vi "Commit DAQ Tags.vi"(8 "error in (no error)":errorcluster, 11 "DAQ State in":T1) -> (0 "error out":errorcluster, 3 "DAQ State out":T1)   [LabVIEW 2018, in "DAQ.lvlib" / "DAQ Write.lvlib"]
uses:
  DAQ Write.lvlib
  Acquisition/Hardware Configuration.ctl
  Acquisition/Task Cluster.ctl
  Tag VIs/Tag FGV Operation Enum.ctl
  Shared Variables/Dynamic Shared Variables.lvlib
  <resource>/objmgr/daqmx.rc
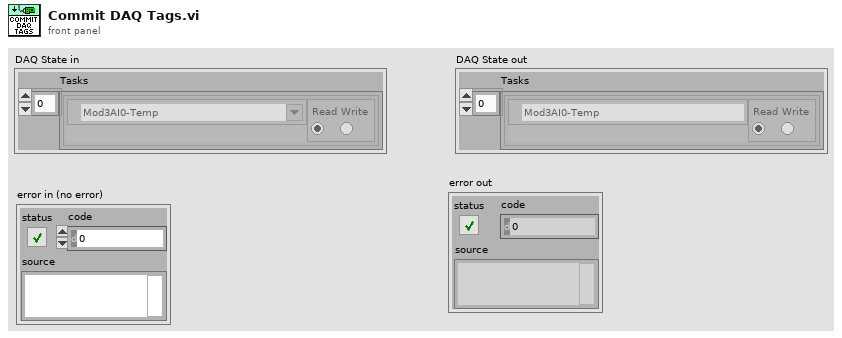
[diagram p1: front panel]
types:
  T1 = typedef "DAQ.lvlib/DAQ Write.lvlib/Hardware Configuration.ctl" = cluster{"Tasks":T2[]}
  T2 = typedef "Task Cluster.ctl" = cluster{"DAQmx Task":refnum<k21>, "Read-Write Radio":enum32{"Read", "Write"}}
  T3 = typedef "Tag FGV Operation Enum.ctl" = enum16{"Init", "Set Notification Queue", "Create Tag", "Commit", "Write Tag (Numeric)", "Write Tag (Boolean)", "Read All Tags", "Read One Tag", "Delete Tag Category", "Set Alarm Parameters (Numeric)", "Set Alarm Parameters (Boolean)", "Enable All Alarms", "Disable All Alarms", "Delete All Tags", "Read Alarms", "Ack Alarm", "Read Alarm Parameters (Numeric)", "Read Alarm Parameters (Boolean)"}
  T4 = enum32{"u32BitField", "bool", "double", "string", "int8", "uint8", "int16", "uint16", "int32", "uint32", "int64", "uint64", "single", "double waveform", "int16 waveform", "array of boolean", "array of int8", "array of uint8", "array of int16", "array of uint16", "array of int32", "array of uint32", "array of int64", "array of uint64", "array of single", "array of double", "array of double waveform", "array of int16 waveform", "array of string", "variant", "timestamp", "fixed point", "custom"}
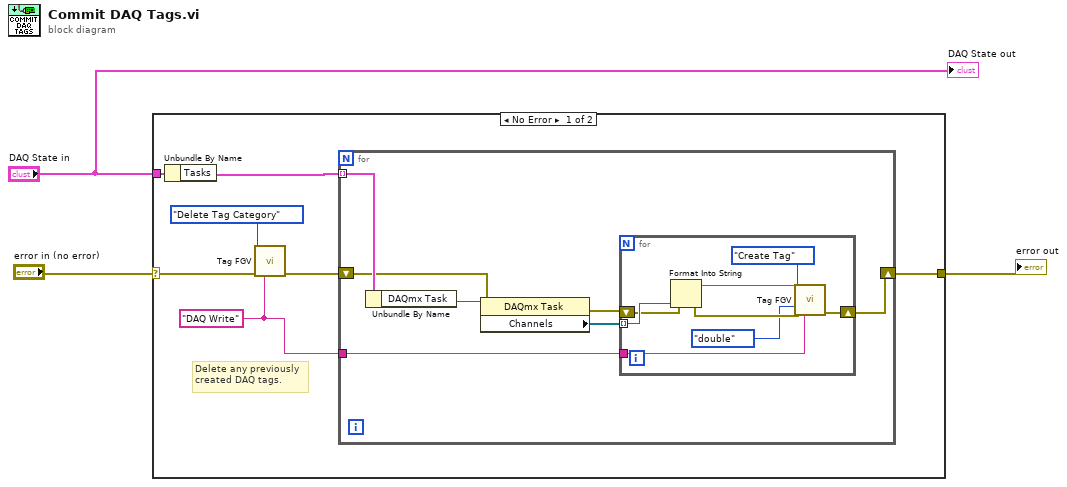
[diagram p0: block diagram]
diagram:
  n1 = case shown="No Error" "error in (no error)" {
    selector: "error in (no error)" -> [w6 w26]
    tunnel: "DAQ State in" -> [w9 _]
    tunnel: [w8 w26] -> w1
    frame No Error {
      w4 = "DAQ Write" ("Tag Category")
      # "Delete any previously\ncreated DAQ tags."
      n2 = Unbundle By Name(w9) -> ("Tasks"=w10:T2[])
      n3 = call "Tag FGV.vi"("Operation"=Tag_FGV_Operation_Enum."Delete Tag Category", "error in (no error)"=w6, "Tag Category"=w4) -> ("error out"=w5:errorcluster)  [unwired: 5 in, 7 out]
      n4 = for {
        tunnel: w10 -> [w13] mode=indexing
        shift-right: [w17] -> w8
        shift-left: w5 -> [w12]
        tunnel: w4 -> [w11]
        n5 = Unbundle By Name(w13) -> ("DAQmx Task"=w14:refnum<k21>)
        n6 = property class="DAQmx Task"(reference=w14, error in=w12) -> (error out=w16:errorcluster, "Channels"=w15:refnum<k21>[])  [unwired: 1 out]
        n7 = for {
          tunnel: w15 -> [w22] mode=indexing
          shift-right: [w25] -> w17
          shift-left: w16 -> [w21]
          tunnel: w11 -> [w19]
          n8 = Format Into String(error in=w21, w22) -> (resulting string=w24:string, error out=w23:errorcluster)  [unwired: 2 in]
          n9 = call "Tag FGV.vi"("Operation"=Tag_FGV_Operation_Enum."Create Tag", "Tag Name"=w24, "Data"=T4."double" ("data type"), "error in (no error)"=w23, "Tag Category"=w19) -> ("error out"=w25:errorcluster)  [unwired: 3 in, 7 out]
        }
      }
    }
    frame Error {
    }
  }
  "error out" <- w1
  "DAQ State out" <- "DAQ State in"
